vi "Relay Control.vi"(6 "Active UUTs":i32[](array[numeric]), 8 "error in (no error)":errorcluster, 9 "Enabled":bool, 10 "Connection":enum16{"All Off", "Programmer", "I2C", "UART"}(ring), 11 "RF Common Tests in":refnum<class "RF Common Tests.lvclass">) -> (0 "error out":errorcluster)   [LabVIEW 2015, in "RF Common Tests.lvclass"]
doc: "Performs Relay control for the RF Multi-Up Testers"
uses:
  RF Common Tests.lvclass
  CBTF Applications/SmartCast Testing/Main/RF Board Test/Application/Application/Class/typedefs/Instrument Selector -- Enum.ctl
  Classes/Instruments/Relay Matrix/Class/Relay Matrix.lvclass
  Classes/Application/Class/Application.lvclass
  Test Class/Test Class.lvclass
  CBTF Applications/SmartCast Testing/Main/RF Board Test/Application/Application/Class/RF Board Test.lvclass
panel:
  in  "Route Name":string
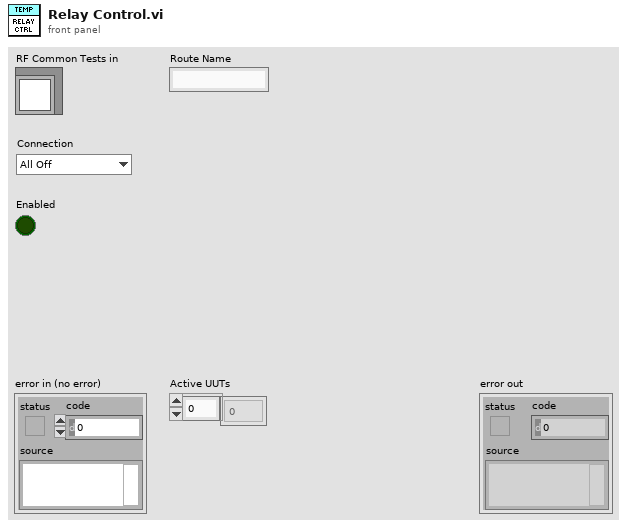
[diagram p1: front panel]
types:
  T1 = typedef "RF Board Test.lvlib/RF Board Test.lvclass/Instrument Selector -- Enum.ctl" = enum16{"RelayMatrix", "MIODevice1", "MIODevice2", "ACPowerSupply", "DCPowerSupply1", "DCPowerSupply2"}
  T2 = typedef "Application.lvlib/App Properties.lvclass/Class Properties -- Cluster.ctl" = cluster{"UUT Info":T3[], "Test Information":refnum<vi>, "Test Complete Event":refnum<user-event>, "Shop Floor System":refnum<class "Shop Floor System.lvclass">, "Gold Board":refnum<class "Golden Board.lvclass">, "Test Recipe":refnum<class "Test Recipe.lvclass">, "Instruments":refnum<class "Instrument.lvclass">[], "Mode":T4, "Test Results":cluster{"Pass":bool[], "Fail Codes":string[]}, "Station Config":refnum<class "Station Config.lvclass">}
  T3 = typedef "Application.lvlib/App Properties.lvclass/UUT Reference -- Cluster.ctl" = cluster{"Serial Number Reference":refnum<vi>, "Status Message Reference":refnum<vi>}
  T4 = typedef "Application.lvlib/Application.lvclass/Op Mode -- Enum.ctl" = u16
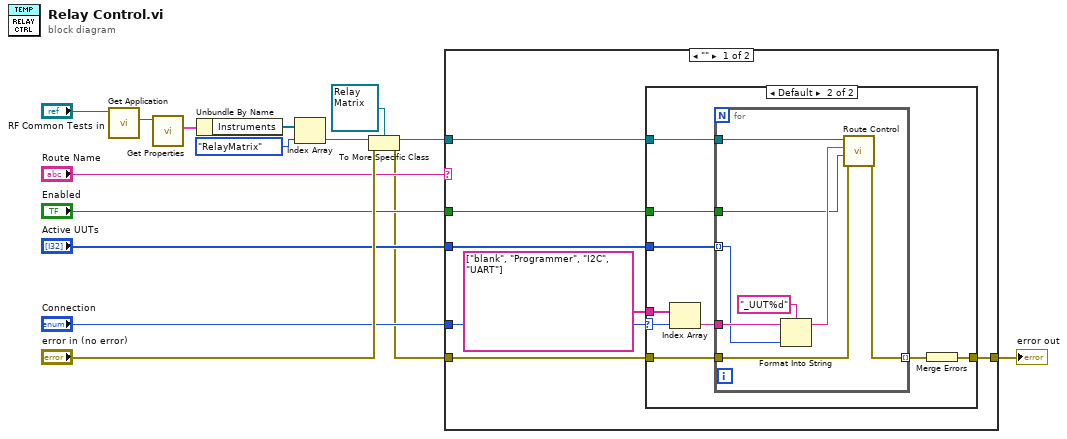
[diagram p0: block diagram]
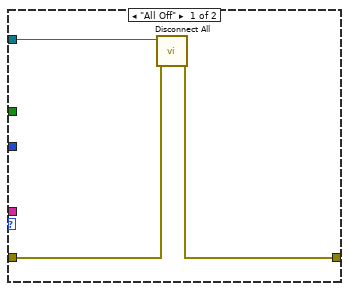
[diagram p2: hidden frame]
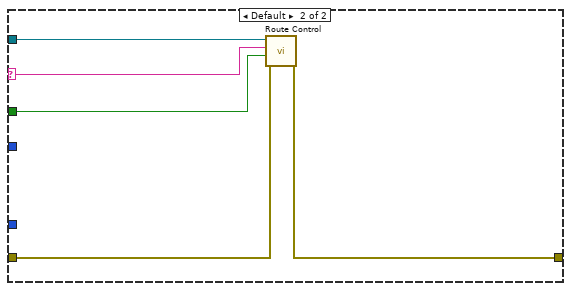
[diagram p3: hidden frame]
diagram:
  n1 = call "Get Application.vi"("Test Class in"="RF Common Tests in") -> ("Application.lvlib:Application.lvclass"=w4:refnum<class "Application.lvclass">)  [unwired: 9 in, 1 out]
  n2 = call "Get Properties.vi"("Acrobat Template in"=w4) -> ("Class Properties"=w5:T2)  [unwired: 8 in, 2 out]
  n3 = Unbundle By Name(w5) -> ("Instruments"=w6:refnum<class "Instrument.lvclass">[])
  n4 = Index Array(array=w6, index=Instrument_Selector_--_Enum."RelayMatrix" ("Instrument")) -> (element=w7:refnum<class "Instrument.lvclass">)
  n5 = To More Specific Class(target class=refnum<class "Relay Matrix.lvclass"> refnum ("Relay Matrix.lvlib:Relay Matrix.lvclass"), reference=w7, error in="error in (no error)") -> (specific class reference=w3:refnum<class "Relay Matrix.lvclass">, error out=w8:errorcluster)
  n6 = case shown="\"\"" "Route Name" {
    selector: "Route Name" -> [_ w45]
    tunnel: w8 -> [w22 w44]
    tunnel: [w21 w43] -> w14
    tunnel: "Connection" -> [w20 _]
    tunnel: "Enabled" -> [w19 w46]
    tunnel: "Active UUTs" -> [w18 _]
    tunnel: w3 -> [w17 w47]
    frame "" {
      n7 = case shown="Default" w20 {
        selector: w20 -> [_ w29]
        tunnel: [w23 w26] -> w21
        tunnel: w22 -> [w24 w31]
        tunnel: w19 -> [_ w33]
        tunnel: w18 -> [_ w34]
        tunnel: w17 -> [w25 w32]
        tunnel: string[] ["blank", "Programmer", "I2C", "UART"] -> [_ w30]
        frame "All Off" {
          n8 = call "Disconnect All.vi"("error in (no error)"=w24, "Acrobat Template in"=w25) -> ("error out"=w23:errorcluster)  [unwired: 8 in, 1 out]
        }
        frame Default {
          n9 = Index Array(array=w30, index=w29) -> (element=w28:string)
          n10 = for {
            tunnel: w34 -> [w41] mode=indexing
            tunnel: w33 -> [w37]
            tunnel: w31 -> [w36]
            tunnel: w28 -> [w42]
            tunnel: [w35] -> w27 mode=indexing
            tunnel: w32 -> [w39]
            n11 = Format Into String(format string="_UUT%d", initial string=w42, w41) -> (resulting string=w38:string)  [unwired: 1 in, 1 out]
            n12 = call "Route Control.vi"("error in (no error)"=w36, "Connect (False)"=w37, "Route Name"=w38, "Acrobat Template in"=w39) -> ("error out"=w35:errorcluster)  [unwired: 6 in, 1 out]
          }
          n13 = Merge Errors(w27) -> (w26:errorcluster)
        }
      }
    }
    frame Default {
      n14 = call "Route Control.vi"("error in (no error)"=w44, "Connect (False)"=w46, "Route Name"=w45, "Acrobat Template in"=w47) -> ("error out"=w43:errorcluster)  [unwired: 6 in, 1 out]
    }
  }
  "error out" <- w14
